vi "Plot Blocks.vi"(0 "picture in":picture, 5 "blocks":T1[](array[typedef]), 12 "pixy resolution":cluster{"width":u16, "height":u16}={"width"=316, "height"=208}, 13 "image resolution":cluster{"width":u16, "height":u16}={"width"=316, "height"=208}) -> (4 "picture out":picture)   [LabVIEW 2018, in "Pixy2.lvlib"]
uses:
  Pixy2.lvlib
  Types/Block.ctl
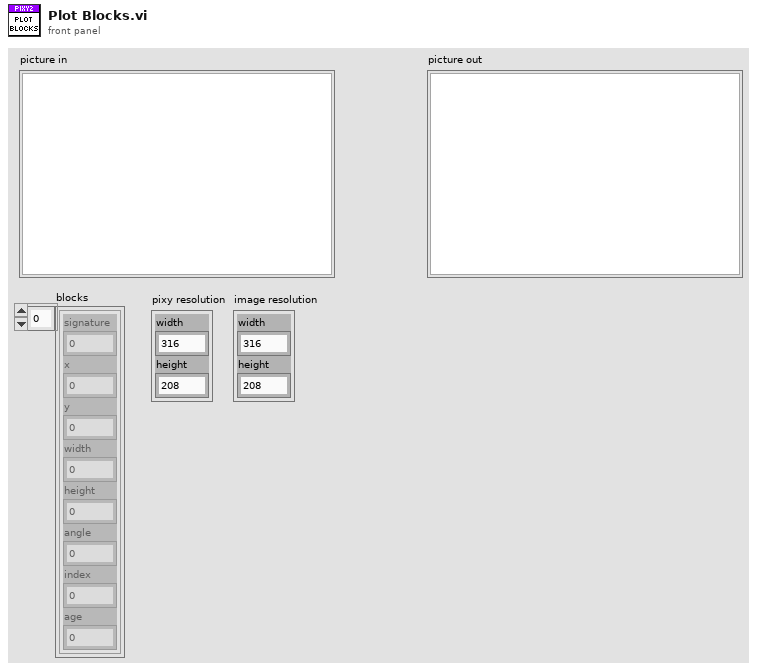
[diagram p1: front panel]
types:
  T1 = typedef "Pixy2.lvlib/Block.ctl" = cluster{"signature":u16, "x":u16, "y":u16, "width":u16, "height":u16, "angle":i16, "index":u8, "age":u8}
  T2 = cluster{"left":i16, "top":i16, "right":i16, "bottom":i16}
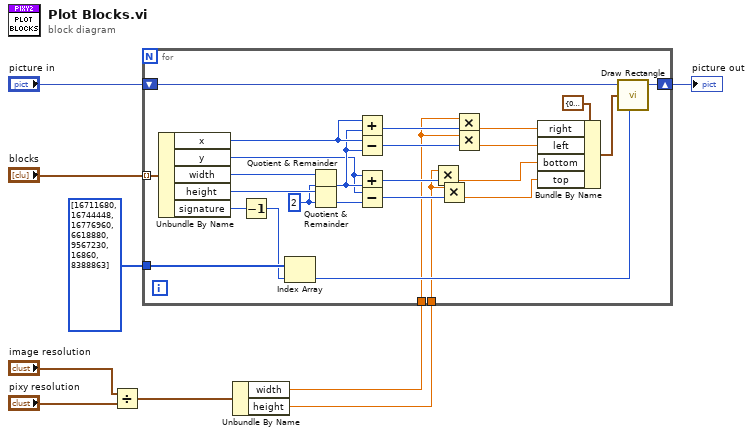
[diagram p0: block diagram]
diagram:
  n1 = Divide(x="image resolution", y="pixy resolution") -> (x/y=w3:cluster{"width":dbl, "height":dbl})
  n2 = Unbundle By Name(w3) -> ("width"=w1:dbl, "height"=w2:dbl)
  n3 = for {
    shift-right: [w35] -> w8
    shift-left: "picture in" -> [w20]
    tunnel: "blocks" -> [w34] mode=indexing
    tunnel: u32[] [16711680, 16744448, 16776960, 6618880, 9567230, 16860, 8388863] -> [w19]
    tunnel: w2 -> [w11]
    tunnel: w1 -> [w10]
    w30 = u16 2 ("y")
    n4 = Unbundle By Name(w34) -> ("x"=w29:u16, "y"=w27:u16, "width"=w31:u16, "height"=w33:u16, "signature"=w18:u16)
    n5 = Decrement(x=w18) -> (x-1=w16:u16)
    n6 = Index Array(array=w19, index=w16) -> (element=w17:u32)
    n7 = Quotient & Remainder(x=w31, y=w30) -> (floor(x/y)=w28:u16)  [unwired: 1 out]
    n8 = Quotient & Remainder(x=w33, y=w30) -> (floor(x/y)=w32:u16)  [unwired: 1 out]
    n9 = Add(x=w29, y=w28) -> (x+y=w24:u16)
    n10 = Subtract(x=w29, y=w28) -> (x-y=w25:u16)
    n11 = Add(x=w27, y=w28) -> (x+y=w22:u16)
    n12 = Subtract(x=w27, y=w32) -> (x-y=w23:u16)
    n13 = Multiply(x=w11, y=w22) -> (x*y=w14:dbl)
    n14 = Multiply(x=w11, y=w23) -> (x*y=w15:dbl)
    n15 = Multiply(x=w10, y=w24) -> (x*y=w12:dbl)
    n16 = Multiply(x=w10, y=w25) -> (x*y=w13:dbl)
    n17 = Bundle By Name(cluster=T2 {"left"=0, "top"=0, "right"=0, "bottom"=0} ("rect"), "right"=w12, "left"=w13, "bottom"=w14, "top"=w15) -> (w21:T2)
    n18 = call <vilib>:"Draw Rectangle.vi"("picture"=w20, "rect"=w21, "color(black)"=w17) -> ("new picture"=w35:picture)  [unwired: 6 in]
  }
  "picture out" <- w8
